vi "filter_2.vi"(10 "data_input":dbl[](array[numeric])) -> (2 "appended array":dbl[][](array[numeric]))   [LabVIEW 2020]
uses:
  <vilib>/Analysis/4window.llb/Parzen Window (DBL).vi
  <vilib>/Analysis/NI_AALPro.lvlib
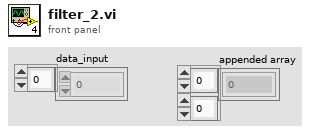
[diagram p1: front panel]
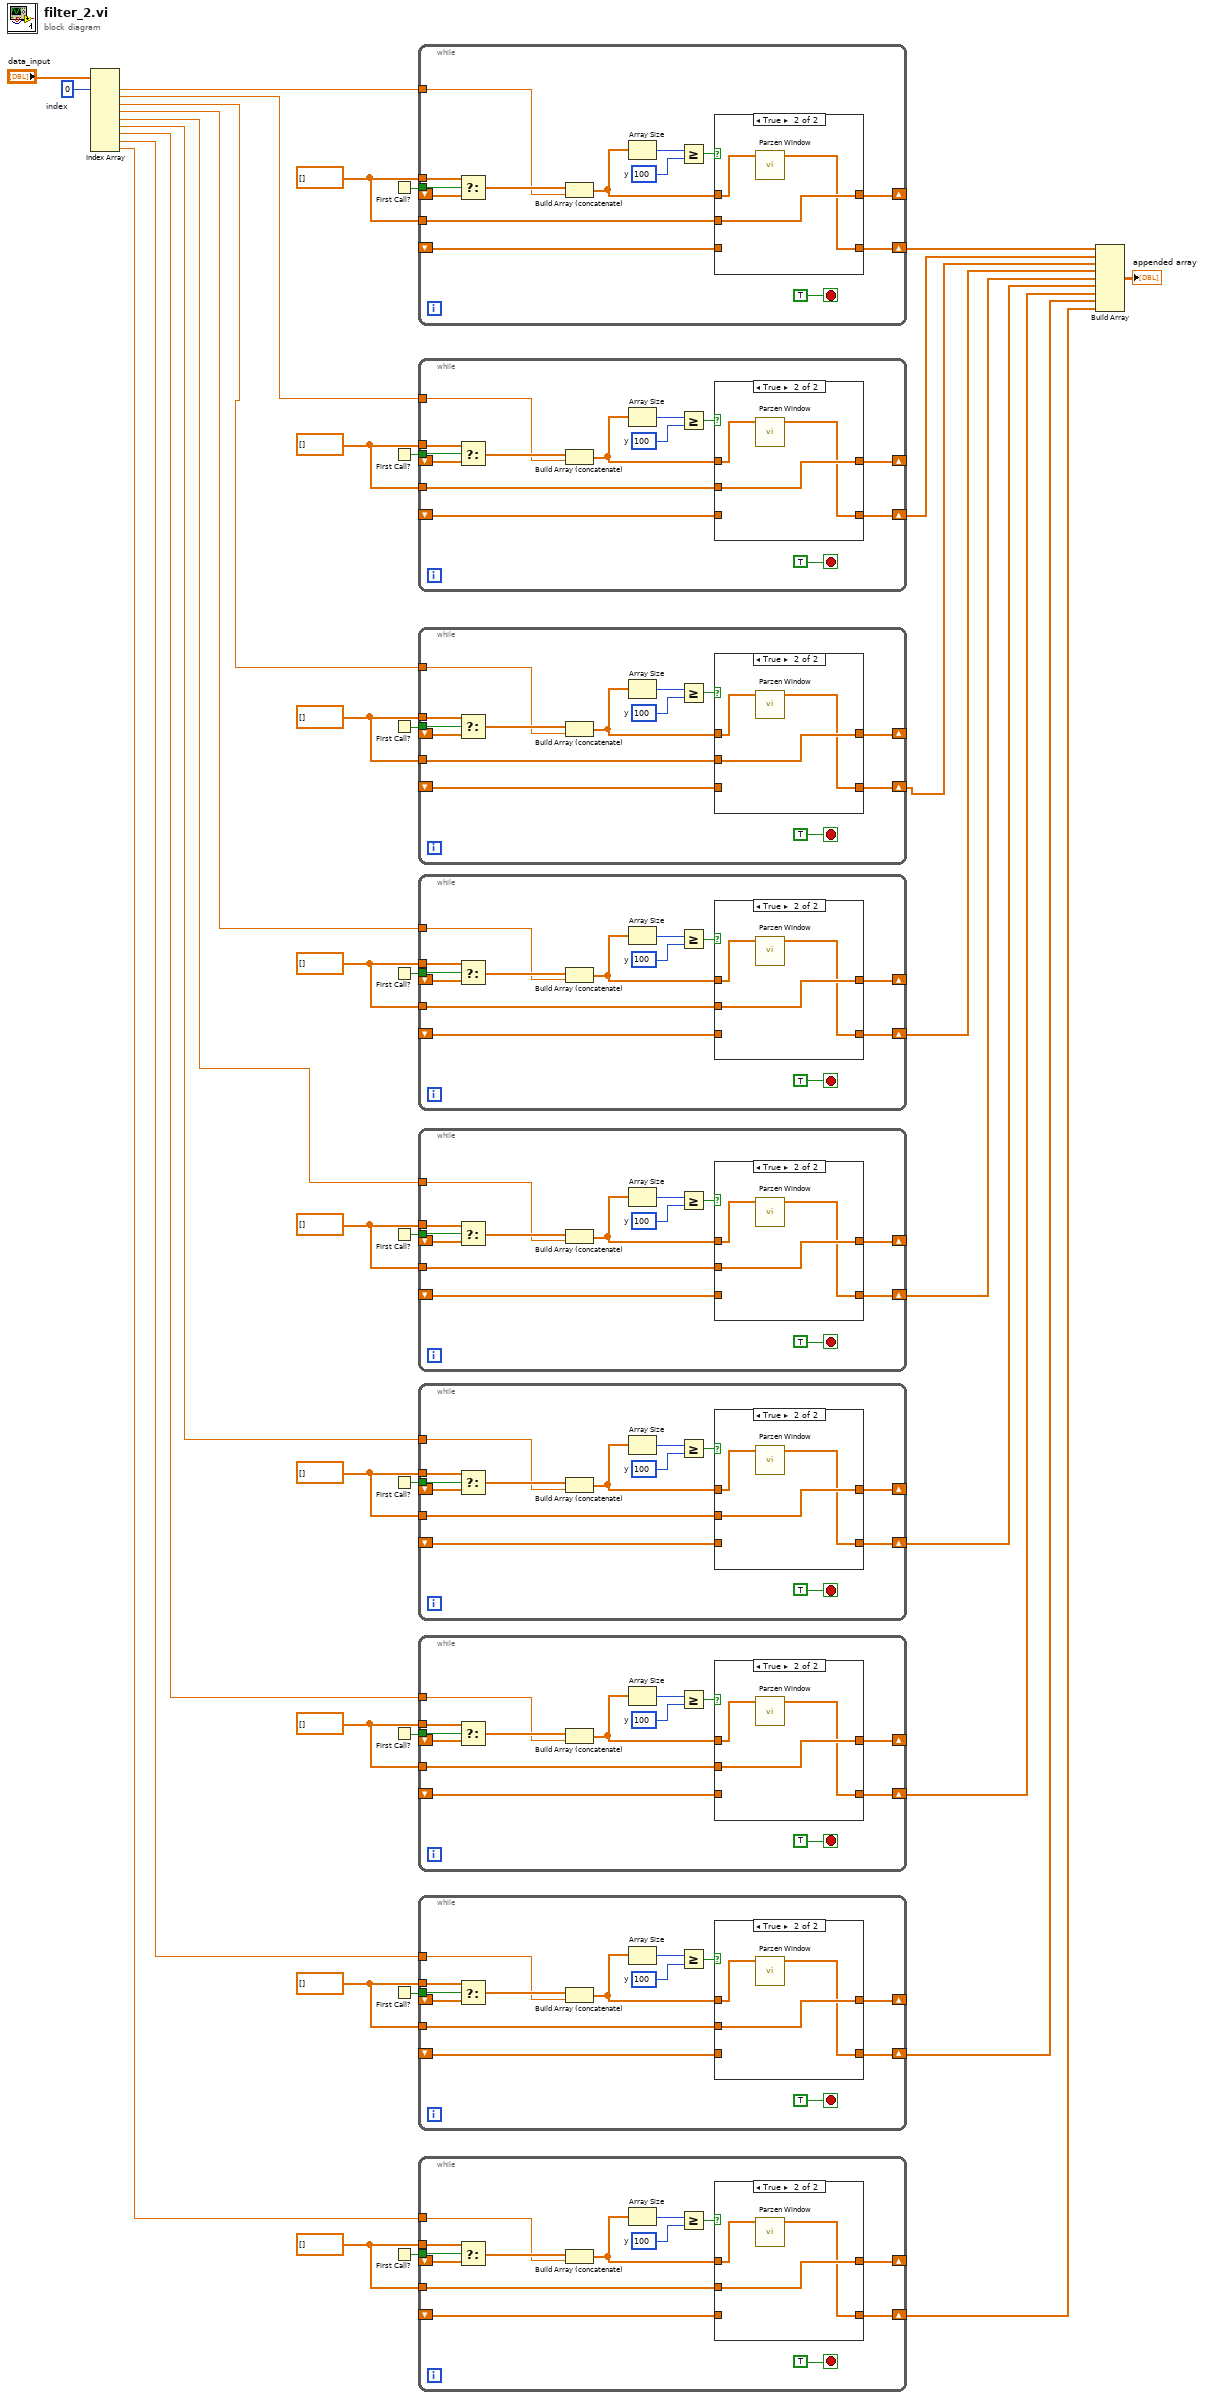
[diagram p0: block diagram]
diagram:
  w13 = dbl[] []
  w16 = dbl[] []
  w19 = dbl[] []
  w22 = dbl[] []
  w27 = dbl[] []
  w30 = dbl[] []
  w31 = dbl[] []
  w34 = dbl[] []
  w35 = dbl[] []
  w39 = 0  # index
  n1 = Index Array(array="data_input", index #1=w39) -> (element #1=w37:dbl, element #2=w26:dbl, element #3=w25:dbl, element #4=w24:dbl, element #5=w23:dbl, element #6=w18:dbl, element #7=w17:dbl, element #8=w12:dbl, element #9=w11:dbl)  [unwired: 8 in]
  n2 = First Call?() -> (First Call?: T/F=w36:bool)
  n3 = First Call?() -> (First Call?: T/F=w33:bool)
  n4 = First Call?() -> (First Call?: T/F=w32:bool)
  n5 = First Call?() -> (First Call?: T/F=w29:bool)
  n6 = First Call?() -> (First Call?: T/F=w28:bool)
  n7 = First Call?() -> (First Call?: T/F=w21:bool)
  n8 = First Call?() -> (First Call?: T/F=w20:bool)
  n9 = First Call?() -> (First Call?: T/F=w15:bool)
  n10 = First Call?() -> (First Call?: T/F=w14:bool)
  n11 = while {
    tunnel: w37 -> [w49]
    tunnel: w36 -> [w51]
    shift-right: [w43] -> _
    shift-left: _ -> [w48]
    tunnel: w35 -> [w52]
    tunnel: w35 -> [w42]
    shift-right: [w41] -> w10
    shift-left: _ -> [w40]
    stop <- TRUE stop-if-true
    w46 = 100  # y
    n12 = Select(t=w52, s=w51, f=w48) -> (s? t:f=w50:dbl[])
    n13 = Build Array (concatenate)(w50, w49) -> (w44:dbl[])
    n14 = Array Size(array=w44) -> (size(s)=w47:i32)
    n15 = Greater Or Equal?(x=w47, y=w46) -> (x >= y?=w45:bool)
    n16 = case shown="True" w45 {
      tunnel: w44 -> [w55 w57]
      tunnel: [w55 w58] -> w43
      tunnel: w42 -> [_ w58]
      tunnel: [w54 w56] -> w41
      tunnel: w40 -> [w54 _]
      frame False {
      }
      frame True {
        n17 = call-poly <vilib>:"Parzen Window.vi"("X"=w57) -> ("Windowed X"=w56:dbl[])  [unwired: 9 in, 1 out]
      }
    }
  }
  n18 = while {
    tunnel: w26 -> [w68]
    tunnel: w33 -> [w70]
    shift-right: [w62] -> _
    shift-left: _ -> [w67]
    tunnel: w34 -> [w71]
    tunnel: w34 -> [w61]
    shift-right: [w60] -> w9
    shift-left: _ -> [w59]
    stop <- TRUE stop-if-true
    w65 = 100  # y
    n19 = Select(t=w71, s=w70, f=w67) -> (s? t:f=w69:dbl[])
    n20 = Build Array (concatenate)(w69, w68) -> (w63:dbl[])
    n21 = Array Size(array=w63) -> (size(s)=w66:i32)
    n22 = Greater Or Equal?(x=w66, y=w65) -> (x >= y?=w64:bool)
    n23 = case shown="True" w64 {
      tunnel: w63 -> [w74 w76]
      tunnel: [w74 w77] -> w62
      tunnel: w61 -> [_ w77]
      tunnel: [w73 w75] -> w60
      tunnel: w59 -> [w73 _]
      frame False {
      }
      frame True {
        n24 = call-poly <vilib>:"Parzen Window.vi"("X"=w76) -> ("Windowed X"=w75:dbl[])  [unwired: 9 in, 1 out]
      }
    }
  }
  n25 = while {
    tunnel: w25 -> [w87]
    tunnel: w32 -> [w89]
    shift-right: [w81] -> _
    shift-left: _ -> [w86]
    tunnel: w31 -> [w90]
    tunnel: w31 -> [w80]
    shift-right: [w79] -> w8
    shift-left: _ -> [w78]
    stop <- TRUE stop-if-true
    w84 = 100  # y
    n26 = Select(t=w90, s=w89, f=w86) -> (s? t:f=w88:dbl[])
    n27 = Build Array (concatenate)(w88, w87) -> (w82:dbl[])
    n28 = Array Size(array=w82) -> (size(s)=w85:i32)
    n29 = Greater Or Equal?(x=w85, y=w84) -> (x >= y?=w83:bool)
    n30 = case shown="True" w83 {
      tunnel: w82 -> [w93 w95]
      tunnel: [w93 w96] -> w81
      tunnel: w80 -> [_ w96]
      tunnel: [w92 w94] -> w79
      tunnel: w78 -> [w92 _]
      frame False {
      }
      frame True {
        n31 = call-poly <vilib>:"Parzen Window.vi"("X"=w95) -> ("Windowed X"=w94:dbl[])  [unwired: 9 in, 1 out]
      }
    }
  }
  n32 = while {
    tunnel: w24 -> [w106]
    tunnel: w29 -> [w108]
    shift-right: [w100] -> _
    shift-left: _ -> [w105]
    tunnel: w30 -> [w109]
    tunnel: w30 -> [w99]
    shift-right: [w98] -> w7
    shift-left: _ -> [w97]
    stop <- TRUE stop-if-true
    w103 = 100  # y
    n33 = Select(t=w109, s=w108, f=w105) -> (s? t:f=w107:dbl[])
    n34 = Build Array (concatenate)(w107, w106) -> (w101:dbl[])
    n35 = Array Size(array=w101) -> (size(s)=w104:i32)
    n36 = Greater Or Equal?(x=w104, y=w103) -> (x >= y?=w102:bool)
    n37 = case shown="True" w102 {
      tunnel: w101 -> [w112 w114]
      tunnel: [w112 w115] -> w100
      tunnel: w99 -> [_ w115]
      tunnel: [w111 w113] -> w98
      tunnel: w97 -> [w111 _]
      frame False {
      }
      frame True {
        n38 = call-poly <vilib>:"Parzen Window.vi"("X"=w114) -> ("Windowed X"=w113:dbl[])  [unwired: 9 in, 1 out]
      }
    }
  }
  n39 = while {
    tunnel: w23 -> [w125]
    tunnel: w28 -> [w127]
    shift-right: [w119] -> _
    shift-left: _ -> [w124]
    tunnel: w27 -> [w128]
    tunnel: w27 -> [w118]
    shift-right: [w117] -> w6
    shift-left: _ -> [w116]
    stop <- TRUE stop-if-true
    w122 = 100  # y
    n40 = Select(t=w128, s=w127, f=w124) -> (s? t:f=w126:dbl[])
    n41 = Build Array (concatenate)(w126, w125) -> (w120:dbl[])
    n42 = Array Size(array=w120) -> (size(s)=w123:i32)
    n43 = Greater Or Equal?(x=w123, y=w122) -> (x >= y?=w121:bool)
    n44 = case shown="True" w121 {
      tunnel: w120 -> [w131 w133]
      tunnel: [w131 w134] -> w119
      tunnel: w118 -> [_ w134]
      tunnel: [w130 w132] -> w117
      tunnel: w116 -> [w130 _]
      frame False {
      }
      frame True {
        n45 = call-poly <vilib>:"Parzen Window.vi"("X"=w133) -> ("Windowed X"=w132:dbl[])  [unwired: 9 in, 1 out]
      }
    }
  }
  n46 = while {
    tunnel: w18 -> [w144]
    tunnel: w21 -> [w146]
    shift-right: [w138] -> _
    shift-left: _ -> [w143]
    tunnel: w22 -> [w147]
    tunnel: w22 -> [w137]
    shift-right: [w136] -> w5
    shift-left: _ -> [w135]
    stop <- TRUE stop-if-true
    w141 = 100  # y
    n47 = Select(t=w147, s=w146, f=w143) -> (s? t:f=w145:dbl[])
    n48 = Build Array (concatenate)(w145, w144) -> (w139:dbl[])
    n49 = Array Size(array=w139) -> (size(s)=w142:i32)
    n50 = Greater Or Equal?(x=w142, y=w141) -> (x >= y?=w140:bool)
    n51 = case shown="True" w140 {
      tunnel: w139 -> [w150 w152]
      tunnel: [w150 w153] -> w138
      tunnel: w137 -> [_ w153]
      tunnel: [w149 w151] -> w136
      tunnel: w135 -> [w149 _]
      frame False {
      }
      frame True {
        n52 = call-poly <vilib>:"Parzen Window.vi"("X"=w152) -> ("Windowed X"=w151:dbl[])  [unwired: 9 in, 1 out]
      }
    }
  }
  n53 = while {
    tunnel: w17 -> [w163]
    tunnel: w20 -> [w165]
    shift-right: [w157] -> _
    shift-left: _ -> [w162]
    tunnel: w19 -> [w166]
    tunnel: w19 -> [w156]
    shift-right: [w155] -> w4
    shift-left: _ -> [w154]
    stop <- TRUE stop-if-true
    w160 = 100  # y
    n54 = Select(t=w166, s=w165, f=w162) -> (s? t:f=w164:dbl[])
    n55 = Build Array (concatenate)(w164, w163) -> (w158:dbl[])
    n56 = Array Size(array=w158) -> (size(s)=w161:i32)
    n57 = Greater Or Equal?(x=w161, y=w160) -> (x >= y?=w159:bool)
    n58 = case shown="True" w159 {
      tunnel: w158 -> [w169 w171]
      tunnel: [w169 w172] -> w157
      tunnel: w156 -> [_ w172]
      tunnel: [w168 w170] -> w155
      tunnel: w154 -> [w168 _]
      frame False {
      }
      frame True {
        n59 = call-poly <vilib>:"Parzen Window.vi"("X"=w171) -> ("Windowed X"=w170:dbl[])  [unwired: 9 in, 1 out]
      }
    }
  }
  n60 = while {
    tunnel: w12 -> [w182]
    tunnel: w15 -> [w184]
    shift-right: [w176] -> _
    shift-left: _ -> [w181]
    tunnel: w16 -> [w185]
    tunnel: w16 -> [w175]
    shift-right: [w174] -> w3
    shift-left: _ -> [w173]
    stop <- TRUE stop-if-true
    w179 = 100  # y
    n61 = Select(t=w185, s=w184, f=w181) -> (s? t:f=w183:dbl[])
    n62 = Build Array (concatenate)(w183, w182) -> (w177:dbl[])
    n63 = Array Size(array=w177) -> (size(s)=w180:i32)
    n64 = Greater Or Equal?(x=w180, y=w179) -> (x >= y?=w178:bool)
    n65 = case shown="True" w178 {
      tunnel: w177 -> [w188 w190]
      tunnel: [w188 w191] -> w176
      tunnel: w175 -> [_ w191]
      tunnel: [w187 w189] -> w174
      tunnel: w173 -> [w187 _]
      frame False {
      }
      frame True {
        n66 = call-poly <vilib>:"Parzen Window.vi"("X"=w190) -> ("Windowed X"=w189:dbl[])  [unwired: 9 in, 1 out]
      }
    }
  }
  n67 = while {
    tunnel: w11 -> [w201]
    tunnel: w14 -> [w203]
    shift-right: [w195] -> _
    shift-left: _ -> [w200]
    tunnel: w13 -> [w204]
    tunnel: w13 -> [w194]
    shift-right: [w193] -> w2
    shift-left: _ -> [w192]
    stop <- TRUE stop-if-true
    w198 = 100  # y
    n68 = Select(t=w204, s=w203, f=w200) -> (s? t:f=w202:dbl[])
    n69 = Build Array (concatenate)(w202, w201) -> (w196:dbl[])
    n70 = Array Size(array=w196) -> (size(s)=w199:i32)
    n71 = Greater Or Equal?(x=w199, y=w198) -> (x >= y?=w197:bool)
    n72 = case shown="True" w197 {
      tunnel: w196 -> [w207 w209]
      tunnel: [w207 w210] -> w195
      tunnel: w194 -> [_ w210]
      tunnel: [w206 w208] -> w193
      tunnel: w192 -> [w206 _]
      frame False {
      }
      frame True {
        n73 = call-poly <vilib>:"Parzen Window.vi"("X"=w209) -> ("Windowed X"=w208:dbl[])  [unwired: 9 in, 1 out]
      }
    }
  }
  n74 = Build Array(w10, w9, w8, w7, w6, w5, w4, w3, w2) -> (→"appended array":dbl[][])
